vi "Get HW Config File Path.vi"(2 "Reset/Set File Path (F)?":bool, 7 "File Path":path=path "No Path Selected", 11 "Error":errorcluster) -> (8 "File Path":path, 15 "Error":errorcluster)   [LabVIEW 2016]
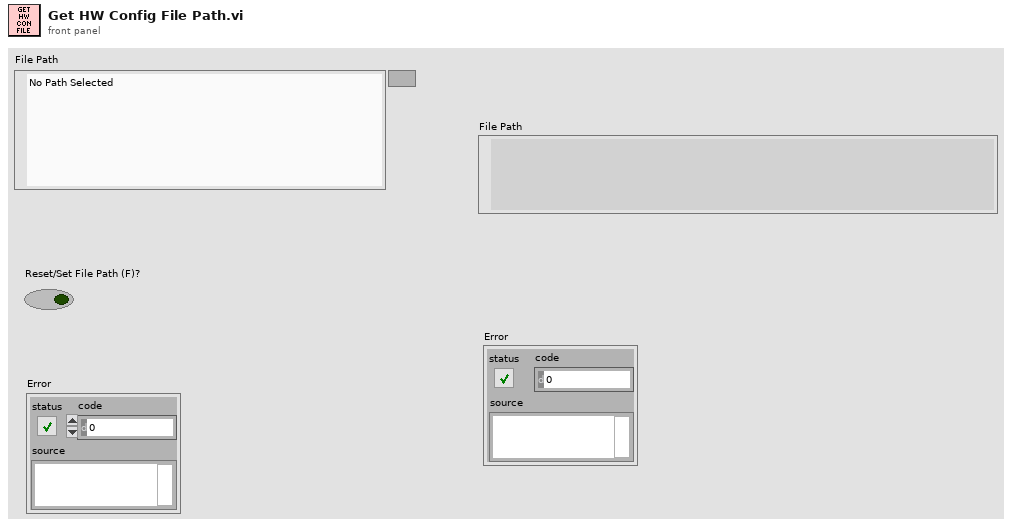
[diagram p1: front panel]
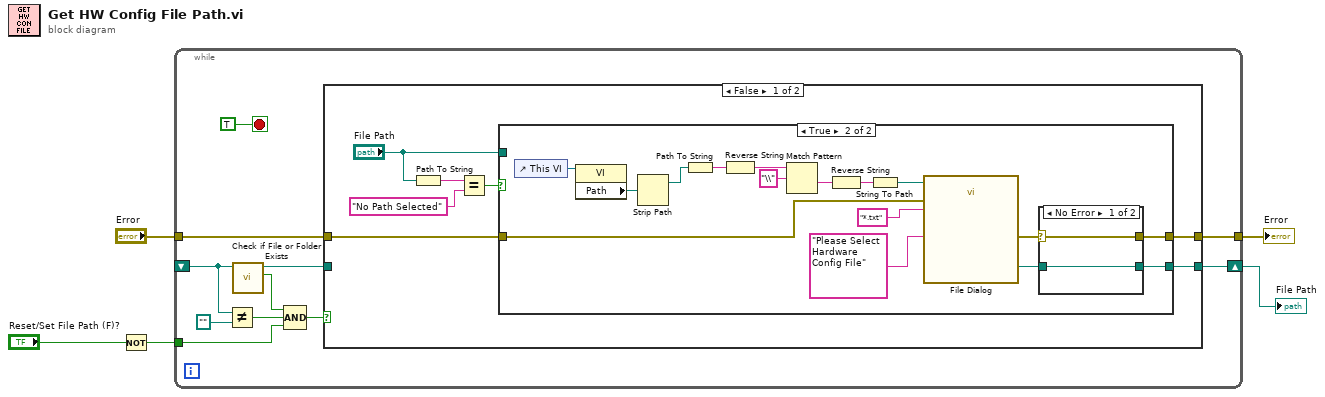
[diagram p0: block diagram]
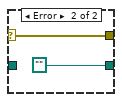
[diagram p3: hidden frame]
diagram:
  n1 = Not(x="Reset/Set File Path (F)?") -> (.not. x?=w2:bool)
  n2 = while {
    shift-right: [w15] -> w5
    shift-left: _ -> [w14]
    tunnel: [w11] -> w4
    tunnel: w2 -> [w8]
    tunnel: "Error" -> [w6]
    stop <- TRUE stop-if-true
    n3 = Not Equal?(x=w14, y=path "") -> (x != y?=w9:bool)
    n4 = call <vilib>:"Check if File or Folder Exists.vi"("path"=w14) -> ("file or folder exists?"=w10:bool, "dup path"=w12:path)  [unwired: 8 in, 1 out]
    n5 = Compound Arithmetic op=AND(w10, w9, w8) -> (w7:bool)
    n6 = case shown="False" w7 {
      tunnel: [w23 w47] -> w15
      tunnel: w12 -> [_ w47]
      tunnel: [w22 w46] -> w11
      tunnel: w6 -> [w17 w46]
      frame False {
        n7 = Path To String(path="File Path") -> (string=w21:string)
        n8 = Equal?(x=w21, y="No Path Selected") -> (x = y?=w19:bool)
        n9 = case shown="True" w19 {
          tunnel: [w25 w35] -> w23
          tunnel: [w24 w34] -> w22
          tunnel: "File Path" -> [w25 _]
          tunnel: w17 -> [w24 w26]
          frame False {
          }
          frame True {
            n10 = control-ref of="This VI"() -> (w40:refnum<vi>)
            n11 = property class="VI"(reference=w40) -> ("Path"=w41:path)  [unwired: 1 in, 2 out]
            n12 = Strip Path(path=w41) -> (stripped path=w27:path)  [unwired: 1 out]
            n13 = Path To String(path=w27) -> (string=w29:string)
            n14 = Reverse String(1:w29) -> (0:w30:string)
            n15 = Match Pattern(string=w30, regular expression="\\") -> (after substring=w32:string)  [unwired: 1 in, 3 out]
            n16 = Reverse String(1:w32) -> (0:w33:string)
            n17 = String To Path(string=w33) -> (path=w28:path)
            n18 = call "File Dialog"("start path"=w28, "prompt"="Please Select Hardware Config File", "error in"=w26, "pattern (all files)"="*.txt") -> ("selected path"=w36:path, "error out"=w37:errorcluster)  [unwired: 8 in, 2 out]
            n19 = case shown="No Error" w37 {
              selector: w37 -> [w42 w44]
              tunnel: w36 -> [w43 _]
              tunnel: [w43 path ""] -> w35
              tunnel: [w42 w44] -> w34
              frame No Error {
              }
              frame Error {
              }
            }
          }
        }
      }
      frame True {
      }
    }
  }
  "File Path" <- w5
  "Error" <- w4
